vi "HMI Loop.vi"(8 "error in (no error)":errorcluster, 11 "device ID in":refnum<k1>) -> (0 "error out":errorcluster, 3 "device ID out":refnum<k1>)   [LabVIEW 2012]
uses:
  <vilib>/Utility/inputDevices.llb/joystickAcquire.vi
panel:
  out "Motor 6":u8(slide) scale=0.0..100.0
  out "UP AND DOWN MOTOR 2":u8(slide) scale=-200.0..200.0
  out "UP AND DOWN MOTOR 1":u8(slide) scale=-200.0..200.0
  out "Speed":u8(slide) scale=-100.0..100.0
  out "Motor 3":u8(slide) scale=0.0..100.0
  out "Motor 4":u8(slide) scale=0.0..100.0
  out "Motor 5":u8(slide) scale=0.0..100.0
  out "direction info":T1
  out "button info":T2
  out "axis info":T3
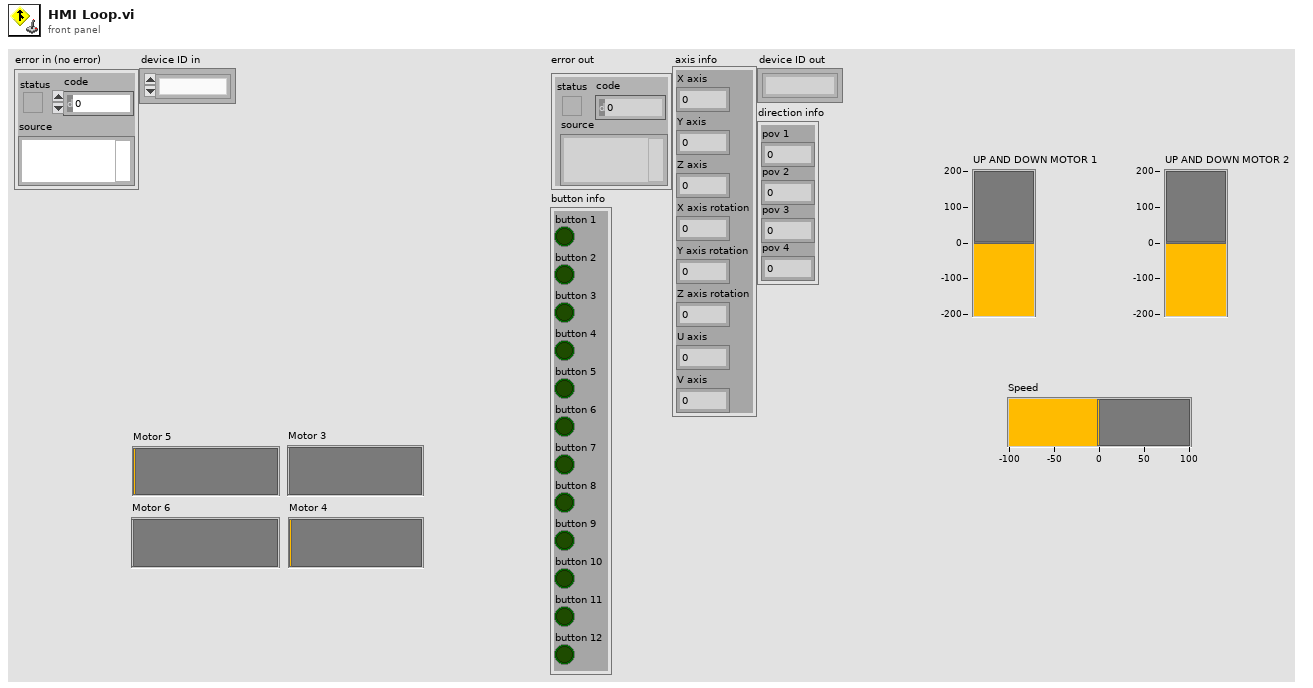
[diagram p1: front panel]
types:
  T1 = cluster{"pov 1":i32, "pov 2":i32, "pov 3":i32, "pov 4":i32}
  T2 = cluster{"button 1":bool, "button 2":bool, "button 3":bool, "button 4":bool, "button 5":bool, "button 6":bool, "button 7":bool, "button 8":bool, "button 9":bool, "button 10":bool, "button 11":bool, "button 12":bool, "button 13":bool, "button 14":bool, "button 15":bool, "button 16":bool, "button 17":bool, "button 18":bool, "button 19":bool, "button 20":bool, "button 21":bool, "button 22":bool, "button 23":bool, "button 24":bool, "button 25":bool, "button 26":bool, "button 27":bool, "button 28":bool, "button 29":bool, "button 30":bool, "button 31":bool, "button 32":bool}
  T3 = cluster{"X axis":i32, "Y axis":i32, "Z axis":i32, "X axis rotation":i32, "Y axis rotation":i32, "Z axis rotation":i32, "U axis":i32, "V axis":i32}
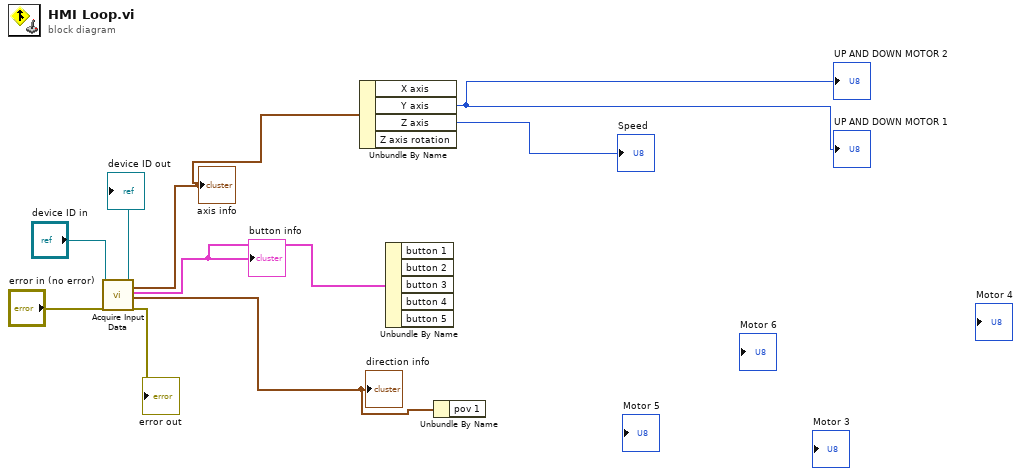
[diagram p0: block diagram]
diagram:
  n1 = call-poly <vilib>:"Acquire Input Data.vi"("device ID"="device ID in", "error in (no error)"="error in (no error)") -> ("device ID"=→"device ID out":refnum<k1>, "axis info"=w3:T3, "button info"=w5:T2, "direction info"=w4:T1, "error out"=→"error out":errorcluster)  [unwired: 13 in]
  "axis info" <- w3
  "button info" <- w5
  "direction info" <- w4
  n2 = Unbundle By Name(w3) -> ("Y axis"=→"UP AND DOWN MOTOR 1" →"UP AND DOWN MOTOR 2":i32, "Z axis"=→"Speed":i32)  [unwired: 2 out]
  n3 = Unbundle By Name(w5) -> ()  [unwired: 5 out]
  n4 = Unbundle By Name(w4) -> ()  [unwired: 1 out]
